vi "XBox Values.vi"(1 "Index":i32 min=0 max=5) -> (0 "XBox":T1)   [LabVIEW 2014]
uses:
  <vilib>/Rock Robotics/Network Tables/SD Write Numeric Array.vi
  <vilib>/Rock Robotics/Network Tables/SD Write Boolean Array.vi
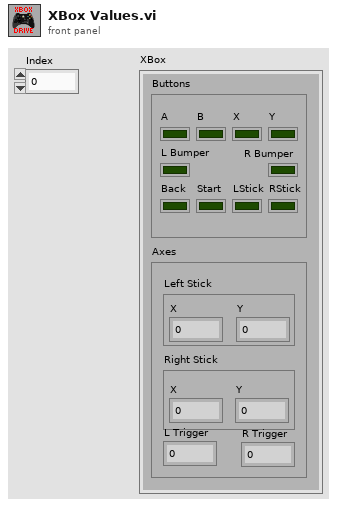
[diagram p1: front panel]
types:
  T1 = cluster{"Buttons":cluster{"A":bool, "B":bool, "X":bool, "Y":bool, "L Bumper":bool, "R Bumper":bool, "Back":bool, "Start":bool, "LStick":bool, "RStick":bool}, "Axes":cluster{"Left Stick":cluster{"X":dbl, "Y":dbl}, "Right Stick":cluster{"X":dbl, "Y":dbl}, "L Trigger":dbl, "R Trigger":dbl}}
  T2 = cluster{"Boolean":bool, "Boolean":bool, "Boolean":bool, "Boolean":bool, "Boolean":bool, "Boolean":bool, "Boolean":bool, "Boolean":bool, "Boolean":bool, "Boolean":bool}
  T3 = cluster{cluster{"Numeric":dbl, "Numeric":dbl}, cluster{"Numeric":dbl, "Numeric":dbl}, "Numeric":dbl, "Numeric":dbl}
  T4 = cluster{cluster{"Boolean":bool, "Boolean":bool, "Boolean":bool, "Boolean":bool, "Boolean":bool, "Boolean":bool, "Boolean":bool, "Boolean":bool, "Boolean":bool, "Boolean":bool}, cluster{cluster{"Numeric":dbl, "Numeric":dbl}, cluster{"Numeric":dbl, "Numeric":dbl}, "Numeric":dbl, "Numeric":dbl}}
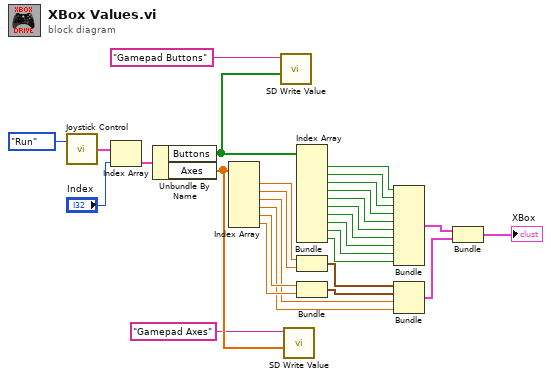
[diagram p0: block diagram]
diagram:
  n1 = call "Joystick Control.vi"("Mode"=enum8{"Start", "Run", "Finish"}."Run") -> ("Joysticks"=w7:cluster{"Buttons":bool[], "Axes":dbl[]}[])  [unwired: 1 in]
  n2 = Index Array(array=w7, index="Index") -> (element=w8:cluster{"Buttons":bool[], "Axes":dbl[]})
  n3 = Unbundle By Name(w8) -> ("Buttons"=w5:bool[], "Axes"=w3:dbl[])
  n4 = Index Array(array=w3) -> (element #1=w19:dbl, element #2=w18:dbl, element #3=w11:dbl, element #4=w10:dbl, element #5=w13:dbl, element #6=w12:dbl)  [unwired: 6 in]
  n5 = call-poly <vilib>:"SD Write Value.vi"("Boolean Array"=w5, "Name"="Gamepad Buttons") -> ()  [unwired: 8 in, 2 out]
  n6 = call-poly <vilib>:"SD Write Value.vi"("Numeric Array"=w3, "Name"="Gamepad Axes") -> ()  [unwired: 8 in, 2 out]
  n7 = Index Array(array=w5) -> (element #1=w29:bool, element #2=w28:bool, element #3=w27:bool, element #4=w25:bool, element #5=w26:bool, element #6=w24:bool, element #7=w23:bool, element #8=w21:bool, element #9=w22:bool, element #10=w20:bool)  [unwired: 10 in]
  n8 = Bundle("Numeric"=w19, "Numeric"=w18) -> (w17:cluster{"Numeric":dbl, "Numeric":dbl})  [unwired: 1 in]
  n9 = Bundle("Numeric"=w13, "Numeric"=w12) -> (w16:cluster{"Numeric":dbl, "Numeric":dbl})  [unwired: 1 in]
  n10 = Bundle("Boolean"=w29, "Boolean"=w28, "Boolean"=w27, "Boolean"=w25, "Boolean"=w26, "Boolean"=w24, "Boolean"=w23, "Boolean"=w21, "Boolean"=w22, "Boolean"=w20) -> (w15:T2)  [unwired: 1 in]
  n11 = Bundle(w17, w16, "Numeric"=w11, "Numeric"=w10) -> (w14:T3)  [unwired: 1 in]
  n12 = Bundle(w15, w14) -> (→"XBox":T4)  [unwired: 1 in]
